vi "Beam_Status.vi"(1 "Power":bool, 4 "Activate":bool, 6 "String":string, 7 "String 3":string, 8 "String 2":string, 9 "String 4":string) -> (10 "?":string, 11 "?":string, 12 "?":string, 13 "?":string, 14 "?":bool, 16 "?":bool, 17 "?":bool, 19 "?":bool)   [LabVIEW 2018, in "com.insstat.lvlib"]
uses:
  com.insstat.lvlib
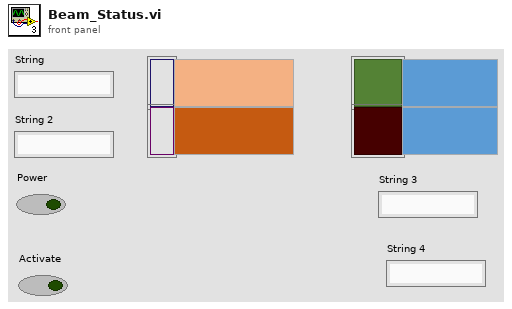
[diagram p1: front panel]
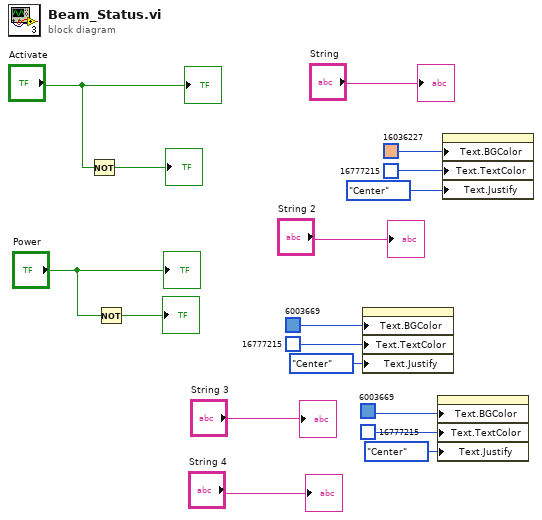
[diagram p0: block diagram]
diagram:
  n1 = Not(x="Activate") -> (.not. x?=→"?":bool)
  n2 = Not(x="Power") -> (.not. x?=→"?":bool)
  n3 = property class="Str"("Text.BGColor"=u32 6003669, "Text.TextColor"=u32 16777215, "Text.Justify"=enum16{"Left", "Center", "Right"}."Center" ("Text.Justification")) -> ()  [unwired: 2 in, 2 out]
  n4 = property class="Str"("Text.BGColor"=u32 6003669, "Text.TextColor"=u32 16777215, "Text.Justify"=enum16{"Left", "Center", "Right"}."Center" ("Text.Justification")) -> ()  [unwired: 2 in, 2 out]
  n5 = property class="Str"("Text.BGColor"=u32 16036227, "Text.TextColor"=u32 16777215, "Text.Justify"=enum16{"Left", "Center", "Right"}."Center" ("Text.Justification")) -> ()  [unwired: 2 in, 2 out]
  "?" <- "Activate"
  "?" <- "String"
  "?" <- "String 2"
  "?" <- "Power"
  "?" <- "String 3"
  "?" <- "String 4"
